vi "Remove Zeroes.vi"(8 "error in (no error)":errorcluster, 11 "Sorted Calibration Points":T1[][](array[typedef])) -> (0 "error out":errorcluster, 3 "Zeroed Out Calibration Points":T1[][](array[typedef]))   [LabVIEW 2026, in "Analysis.lvlib"]
uses:
  controls/Messaging Payloads/Calibration Point Table Insert.ctl
  Analysis.lvlib
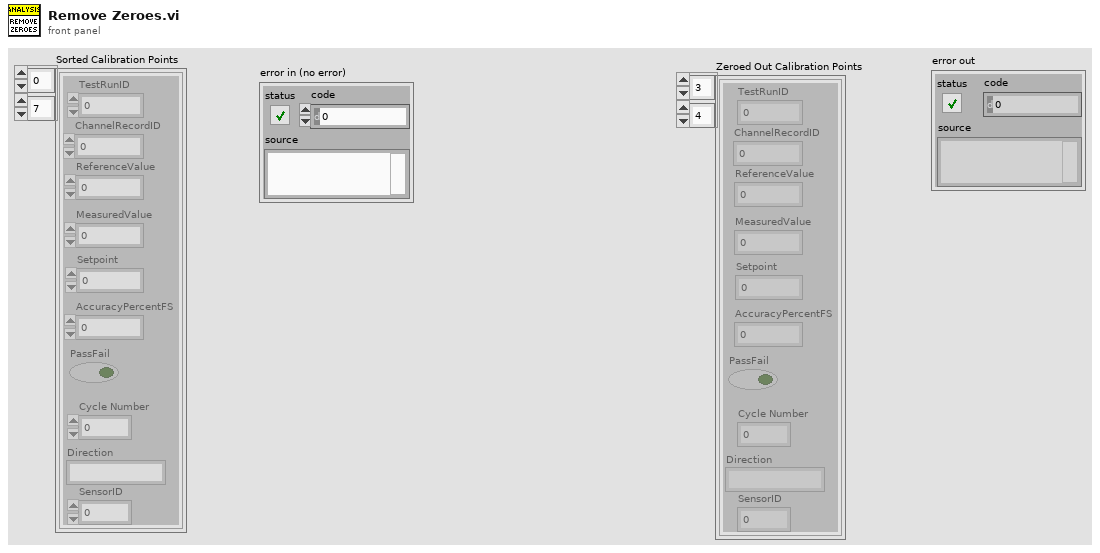
[diagram p1: front panel]
types:
  T1 = typedef "Calibration Point Table Insert.ctl" = cluster{"TestRunID":i32, "ChannelRecordID":i32, "Setpoint":dbl, "MeasuredValue":dbl, "AccuracyPercentFS":dbl, "PassFail":bool, "ReferenceValue":dbl, "Cycle Number":i32, "Direction":string, "SensorID":i32}
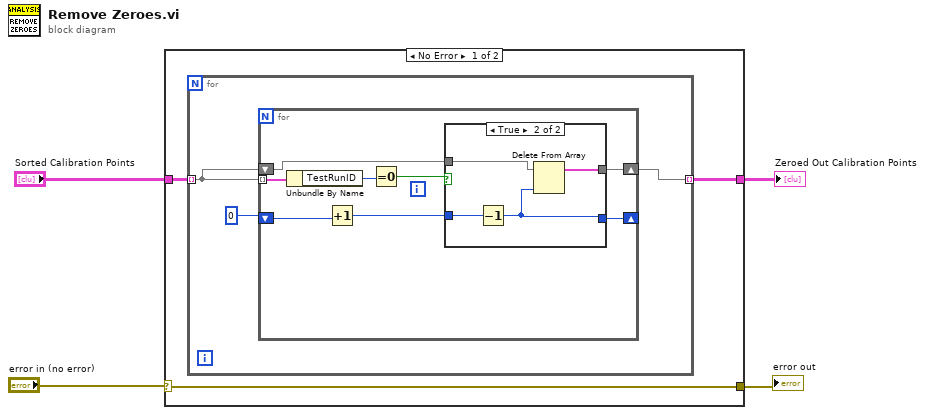
[diagram p0: block diagram]
diagram:
  n1 = case shown="No Error" "error in (no error)" {
    selector: "error in (no error)" -> [w5 w26]
    tunnel: "Sorted Calibration Points" -> [w7 w25]
    tunnel: [w6 w25] -> w3
    tunnel: [w5 w26] -> w1
    frame No Error {
      n2 = for {
        tunnel: w7 -> [w10] mode=indexing
        tunnel: [w9] -> w6 mode=indexing
        n3 = for {
          tunnel: w10 -> [w18] mode=indexing
          shift-right: [w14] -> w9
          shift-left: w10 -> [w15]
          shift-right: [w13] -> _
          shift-left: 0 -> [w12]
          n4 = Unbundle By Name(w18) -> ("TestRunID"=w17:i32)
          n5 = Increment(x=w12) -> (x+1=w11:i32)
          n6 = Equal To 0?(x=w17) -> (x = 0?=w16:bool)
          n7 = case shown="True" w16 {
            tunnel: w15 -> [w20 w24]
            tunnel: [w20 w23] -> w14
            tunnel: [w19 w21] -> w13
            tunnel: w11 -> [w19 w22]
            frame False {
            }
            frame True {
              n8 = Decrement(x=w22) -> (x-1=w21:i32)
              n9 = Delete From Array(array=w24, index=w21) -> (array with subset deleted=w23:T1[])  [unwired: 1 in, 1 out]
            }
          }
        }
      }
    }
    frame Error {
    }
  }
  "Zeroed Out Calibration Points" <- w3
  "error out" <- w1
